vi "NavX.vi"() -> ()   [LabVIEW 2020]
uses:
  <vilib>/High Genius/HG_WSI_Tookit/Dependencies/Library/IMU/IMU.lvclass
  C:/Program Files (x86)/National Instruments/LabVIEW 2020/vi.lib/High Genius/HG_WSI_Tookit/Dependencies/Library/HG_LIB/HG_LIB.lvclass
  <vilib>/Platform/TimedLoop/XDataNode/timing_clust.ctl
  <vilib>/Platform/TimedLoop/XDataNode/nitl_modes.ctl
  <vilib>/Platform/TimedLoop/XDataNode/wakeup.ctl
  <vilib>/platform/TimedLoop/XDataNode/XDataNode.xnode
  <vilib>/High Genius/HG_WSI_Tookit/Dependencies/Library/HG_LIB/HG_LIB.lvclass
  <vilib>/Platform/TimedLoop/XDataNode/XDNodeRunTimeDep.lvlib
panel:
  in  "stop":bool
  out "IMU":dbl[](array[numeric])
  out "YAW (rad)":dbl
  in  "Boolean":bool
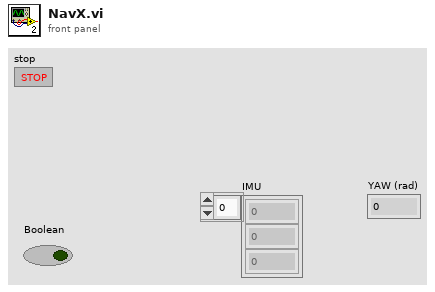
[diagram p1: front panel]
types:
  T1 = enum16{"DI", "DO", "AI", "Pulse", "PWM", "ISQ", "ENC", "CAN", "IIC", "IMU"}
  T2 = typedef "XDNodeRunTimeDep.lvlib/timing_clust.ctl" = cluster{"Expected End [f-1]":u64, "Actual End [f-1]":u64, "Finished Late? [f-1]":bool, "Expected End [i-1]":u64, "Actual End [i-1]":u64, "Finished Late? [i-1]":bool, "Expected Start [i]":u64, "Actual Start [i]":u64, "Expected Start [f]":u64, "Actual Start [f]":u64, "Source Name":string, "Structure Name":string, "Period":i64, "Deadline":i64, "Offset":i64, "Start":i64, "Priority":i32, "Timeout":i32, "Mode":T3, "Wakeup Reason":T4, "Error":errorcluster, "Source Type":string, "Secondary Source Type":string, "Global End Time":u64, "Global Start Time":u64, "Frame Duration":u64, "Iteration Duration":u64, "Assigned CPU":i32, "I/O Scan Engine Mode":u32}
  T3 = typedef "XDNodeRunTimeDep.lvlib/nitl_modes.ctl" = enum32{"No Change", "Process missed periods, maintain original phase", "Discard missed periods, maintain original phase", "Process missed periods, ignore original phase", "Discard missed periods, ignore original phase"}
  T4 = typedef "XDNodeRunTimeDep.lvlib/wakeup.ctl" = enum32{"Normal", "Aborted", "Asynchronous wakeup", "Timing source error", "Timed loop error", "Timeout"}
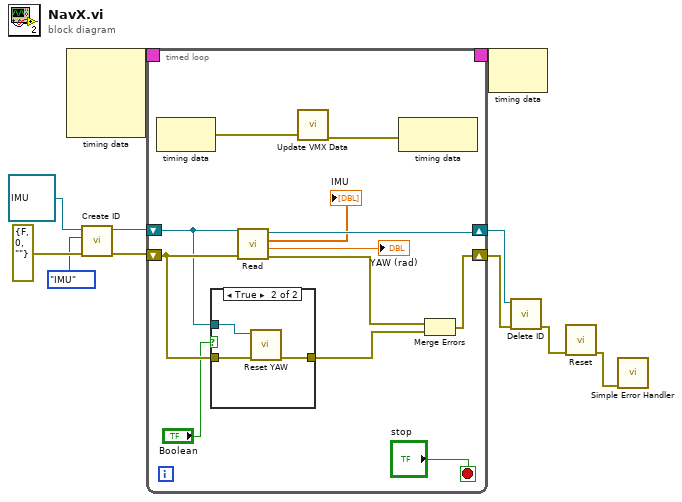
[diagram p0: block diagram]
diagram:
  n1 = node-c288() -> (w4:T2)  [unwired: 4 in]
  n2 = call <vilib>:"Create ID.vi"("error in (no error)"=errorcluster {"status"=FALSE, "code"=0, "source"=""}, "Function"=T1."IMU", "HG_LIB in"=refnum<class "IMU.lvclass"> refnum ("VMX Library.lvlib:IMU.lvclass")) -> ("error out"=w5:errorcluster, "HG_LIB out"=w6:refnum<class "IMU.lvclass">)  [unwired: 7 in]
  n3 = timed-loop {
    timing: w4 -> [_]
    timing-out: [_] -> w3
    shift-right: [w19] -> w1
    shift-left: w6 -> [w18]
    shift-right: [w20] -> w2
    shift-left: w5 -> [w23]
    stop <- "stop" stop-if-true
    n4 = node-c288() -> (w13:errorcluster)  [unwired: 1 in]
    n5 = case shown="True" "Boolean" {
      tunnel: w23 -> [w24 w27]
      tunnel: [w24 w26] -> w22
      tunnel: w18 -> [_ w25]
      frame False {
      }
      frame True {
        n6 = call <vilib>:"Reset YAW.vi"("error in (no error)"=w27, "IMU in"=w25) -> ("error out"=w26:errorcluster)  [unwired: 8 in, 1 out]
      }
    }
    n7 = call <vilib>:"Read.vi"("error in (no error)"=w23, "IMU in"=w18) -> ("error out"=w21:errorcluster, "YAW (rad)"=→"YAW (rad)":dbl, "IMU"=→"IMU":dbl[], "IMU out"=w19:refnum<class "IMU.lvclass">)  [unwired: 6 in]
    n8 = call <vilib>:"Update VMX Data.vi"("error in (no error)"=w13) -> ("error out"=w12:errorcluster)  [unwired: 10 in]
    n9 = node-c288(w12) -> ()  [unwired: 1 out]
    n10 = Merge Errors(w21, w22) -> (w20:errorcluster)
  }
  n11 = node-c288(w3) -> ()  [unwired: 1 out]
  n12 = call <vilib>:"Delete ID.vi"("error in (no error)"=w2, "HG_LIB in"=w1) -> ("error out"=w11:errorcluster)  [unwired: 8 in, 1 out]
  n13 = call <vilib>:"Reset.vi"("error in (no error)"=w11) -> ("error out"=w10:errorcluster)  [unwired: 10 in]
  n14 = call <vilib>:"Simple Error Handler.vi"("error in (no error)"=w10) -> ()  [unwired: 4 in, 5 out]
